vi "SaveArray.vi"(5 "name or relative path":string="test", 7 "saving folder":path=path "D:/Data/Mai/test target/logfile", 8 "error in":errorcluster, 9 "parameters cluster":refnum<vi>[](array[refnum]), 10 "overwrite":bool, 11 "array":dbl[][](array[numeric])) -> (0 "error out":errorcluster)   [LabVIEW 2018, in "RW_Protocols.lvlib"]
uses:
  RW_Protocols.lvlib
panel:
  in  "infos":string
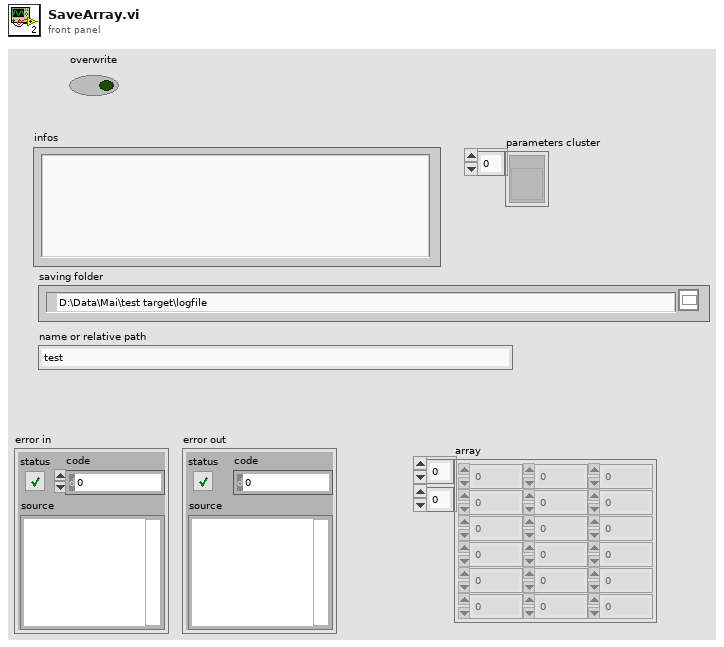
[diagram p1: front panel]
types:
  T1 = enum16{"open", "replace", "create", "open or create", "replace or create", "replace or create with confirmation"}
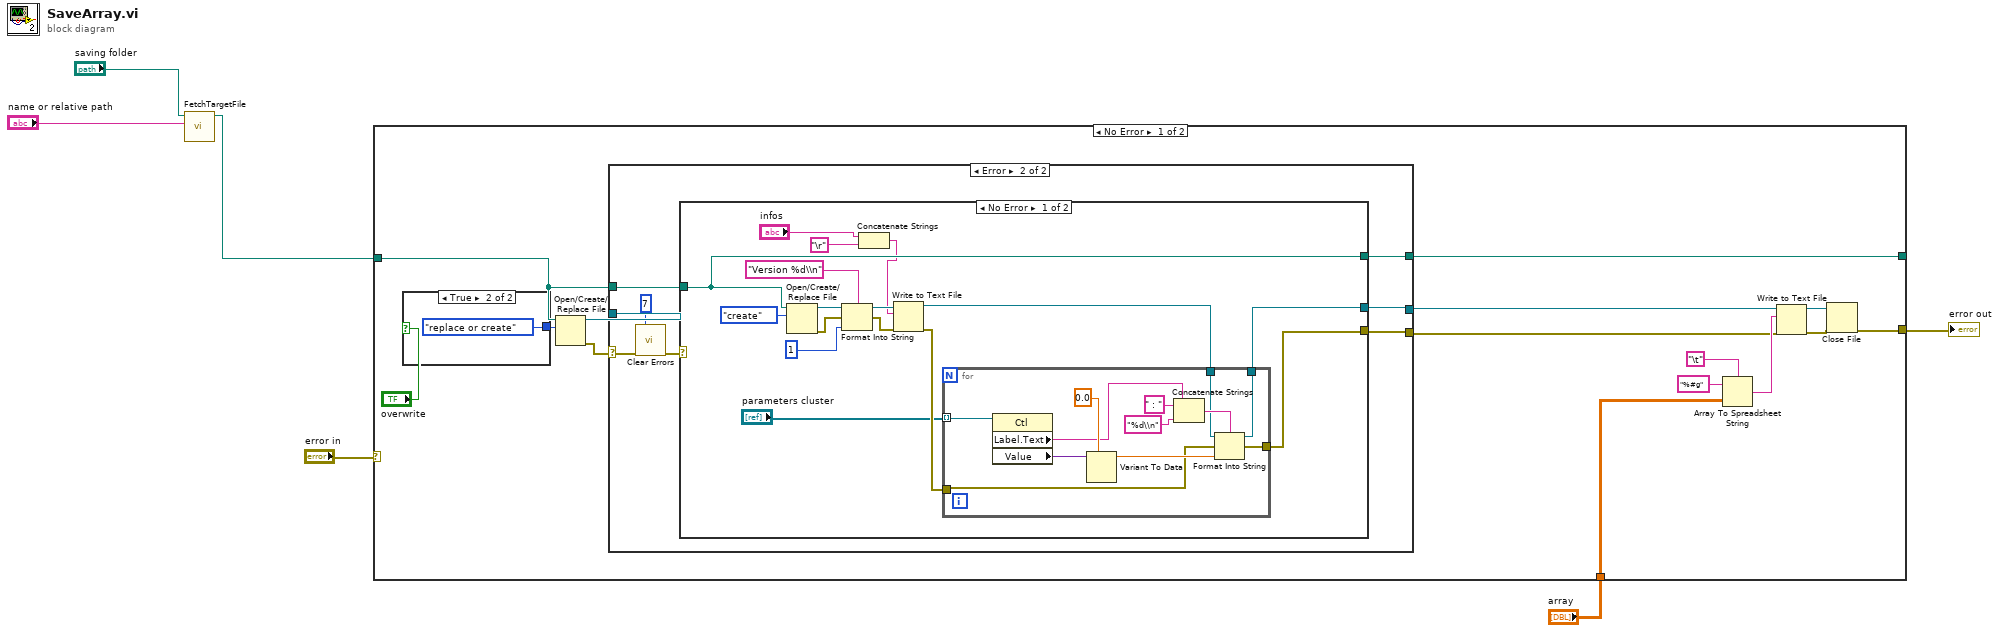
[diagram p0: block diagram]
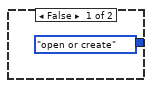
[diagram p2: hidden frame]
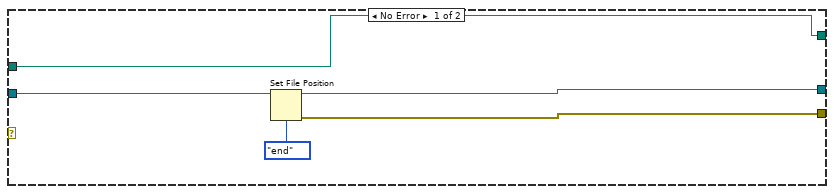
[diagram p3: hidden frame]
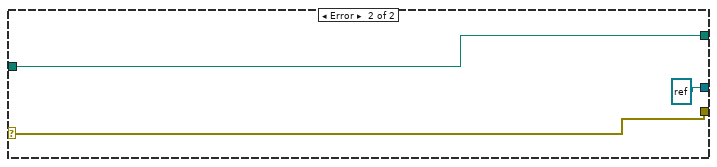
[diagram p4: hidden frame]
diagram:
  n1 = call "FetchTargetFile.vi"("FileName"="name or relative path", "Target Folder"="saving folder") -> ("Full File Path"=w1:path)  [unwired: 8 in, 1 out]
  n2 = case shown="No Error" "error in" {
    selector: "error in" -> [_ w68]
    tunnel: [w17 w68] -> w6
    tunnel: [w20 w67] -> _
    tunnel: w1 -> [w16 w67]
    tunnel: "array" -> [w10 _]
    frame No Error {
      n3 = case shown="True" "overwrite" {
        tunnel: [T1."open or create" ("operation (0:open)") T1."replace or create" ("operation (0:open)")] -> w21
        frame False {
        }
        frame True {
        }
      }
      n4 = Open/Create/Replace File(file path (use dialog)=w16, operation (0:open)=w21) -> (refnum out=w19:refnum<file>, error out=w18:errorcluster)  [unwired: 4 in, 1 out]
      n5 = case shown="Error" w18 {
        selector: w18 -> [_ w34]
        tunnel: [w26 w31] -> w20
        tunnel: w19 -> [w27 _]
        tunnel: w16 -> [w26 w35]
        tunnel: [w24 w29] -> w8
        tunnel: [w25 w30] -> w9
        frame No Error {
          n6 = Set File Position(refnum=w27, from (0:start)=enum16{"start", "end", "current"}."end" ("à partir de (0 : start)")) -> (refnum out=w24:refnum<file>, error out=w25:errorcluster)  [unwired: 2 in]
        }
        frame Error {
          n7 = call <vilib>:"Clear Errors.vi"("error in (no error)"=w34, "specific error code to clear (0: all)"=7) -> ("error out"=w32:errorcluster)  [unwired: 4 in, 1 out]
          n8 = case shown="No Error" w32 {
            selector: w32 -> [_ w65]
            tunnel: w35 -> [w46 w66]
            tunnel: [w46 w66] -> w31
            tunnel: [w37 w65] -> w30
            tunnel: [w36 refnum<file> refnum ("refnum out")] -> w29
            frame No Error {
              n9 = Open/Create/Replace File(file path (use dialog)=w46, operation (0:open)=T1."create") -> (refnum out=w47:refnum<file>, error out=w48:errorcluster)  [unwired: 4 in, 1 out]
              n10 = Format Into String ("Format Into File")(format string="Version %d\\n", initial string=w47, error in=w48, u32 1 ("input 1")) -> (resulting string=w43:refnum<file>, error out=w42:errorcluster)
              n11 = Concatenate Strings("infos", "\r") -> (w39:string)
              n12 = Write to Text File(file (use dialog)=w43, text=w39, error in=w42) -> (refnum out=w44:refnum<file>, error out=w45:errorcluster)  [unwired: 1 in, 1 out]
              n13 = for {
                tunnel: "parameters cluster" -> [w63] mode=indexing
                tunnel: w45 -> [w57]
                tunnel: w44 -> [w56]
                tunnel: [w55] -> w36
                tunnel: [w54] -> w37
                n14 = property class="Ctl"(reference=w63) -> ("Label.Text"=w59:string, "Value"=w62:variant)  [unwired: 1 in, 2 out]
                n15 = Variant To Data(type=0.0, Variant=w62) -> (data=w60:dbl)  [unwired: 1 in, 1 out]
                n16 = Concatenate Strings(w59, " : " ("string"), "%d\\n" ("string")) -> (w58:string)
                n17 = Format Into String ("Format Into File")(format string=w58, initial string=w56, error in=w57, w60) -> (resulting string=w55:refnum<file>, error out=w54:errorcluster)
              }
            }
            frame Error {
            }
          }
        }
      }
      n18 = Array To Spreadsheet String(delimiter (Tab)="\t", array=w10, 3:"%#g" ("format string")) -> (spreadsheet string=w11:string)
      n19 = Write to Text File(file (use dialog)=w8, text=w11, error in=w9) -> (refnum out=w12:refnum<file>, error out=w13:errorcluster)  [unwired: 1 in, 1 out]
      n20 = Close File(refnum=w12, error in=w13) -> (error out=w17:errorcluster)  [unwired: 1 out]
    }
    frame Error {
    }
  }
  "error out" <- w6
